vi "State_Machine.vi"(8 "error in (no error)":errorcluster caption="entrée d'erreur (pas d'erreur)", 11 "Get_Voltage en entrée":refnum<class "P2056_ExitTestBench.lvclass">) -> (0 "error out":errorcluster caption="sortie d'erreur", 2 "Json_String":string, 3 "Get_Voltage en sortie":refnum<class "P2056_ExitTestBench.lvclass">)   [LabVIEW 2020, in "Library Test.lvlib" / "P2056_ExitTestBench.lvclass"]
uses:
  P2056_ExitTestBench.lvclass
  C:/Users/ngarcin/OneDrive - Altyor/Standard TB/Class/Test/P2056_Send_Command_UART/P2056_Send_Command_UART.lvclass
  C:/Users/ngarcin/OneDrive - Altyor/Standard TB/Class/Test/Test (Default)/Test (Default).lvclass
  Instrument/Instrument (Default)/Class Instrument (Default).lvclass
  P2056_ExitTestBench.lvclass/P2056_ExitTestBench.ctl
  P2056_Send_Command_UART/P2056_Send_Command_UART.lvclass
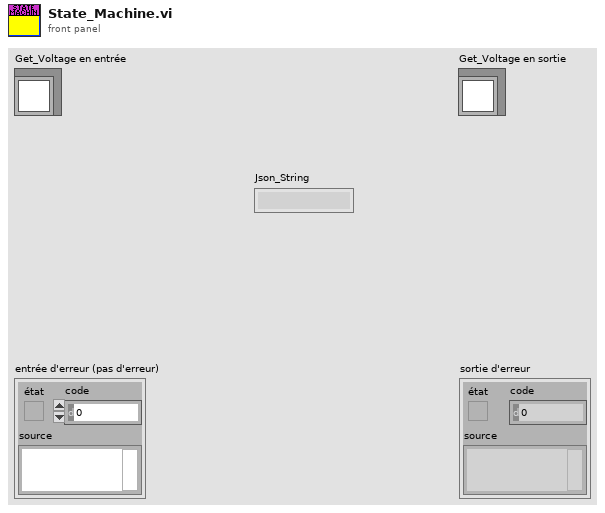
[diagram p1: front panel]
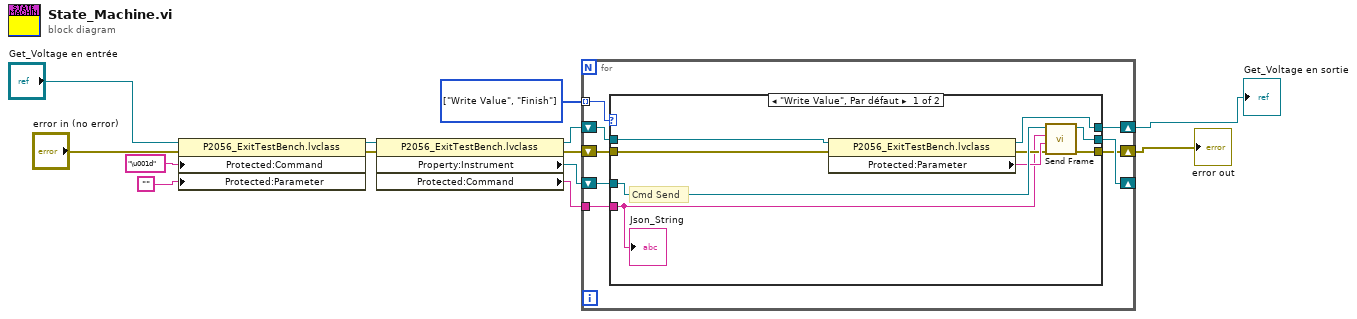
[diagram p0: block diagram]
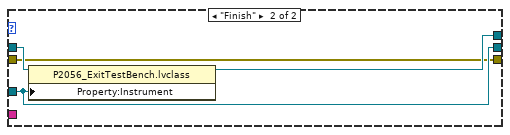
[diagram p2: hidden frame]
diagram:
  w9 = enum16{"Init", "Write Value", "Finish"}[] [enum."Write Value", enum."Finish"] items=["Init", "Write Value", "Finish"]
  n1 = property class="P2056_ExitTestBench.lvclass"(reference="Get_Voltage en entrée", error in="error in (no error)", "Protected:Command"="\u001d" ("chaîne"), "Protected:Parameter"="") -> (reference out=w4:refnum<class "P2056_ExitTestBench.lvclass">, error out=w3:errorcluster)
  n2 = property class="P2056_ExitTestBench.lvclass"(reference=w4, error in=w3) -> (reference out=w7:refnum<class "P2056_ExitTestBench.lvclass">, error out=w6:errorcluster, "Property:Instrument"=w8:refnum<class "Class Instrument (Default).lvclass">, "Protected:Command"=w5:string)
  n3 = for {
    tunnel: w9 -> [w21] mode=indexing
    shift-right: [w19] -> _
    shift-left: w8 -> [w20]
    shift-right: [w17] -> w1
    shift-left: w7 -> [w18]
    shift-right: [w15] -> w2
    shift-left: w6 -> [w16]
    tunnel: w5 -> [w14]
    n4 = case shown="\"Write Value\", Par défaut" w21 {
      tunnel: w20 -> [w28 w32]
      tunnel: [w29 w32] -> w19
      tunnel: w18 -> [w27 w34]
      tunnel: [w26 w33] -> w17
      tunnel: w16 -> [w24 w31]
      tunnel: [w30 w31] -> w15
      tunnel: w14 -> [w22 _]
      frame "Write Value", Default {
        # "Cmd Send"
        n5 = property class="P2056_ExitTestBench.lvclass"(reference=w27, error in=w24) -> (reference out=w26:refnum<class "P2056_ExitTestBench.lvclass">, error out=w23:errorcluster, "Protected:Parameter"=w25:string)
        n6 = call "Send Frame.vi"("entrée d'erreur (pas d'erreur)"=w23, "Parameter"=w25, "Cmd"=w22, "Class Instrument (Default) en entrée"=w28) -> ("sortie d'erreur"=w30:errorcluster, "Class Instrument (Default) en sortie"=w29:refnum<class "Class Instrument (Default).lvclass">)  [unwired: 6 in]
        "Json_String" <- w22
      }
      frame "Finish" {
        n7 = property class="P2056_ExitTestBench.lvclass"(reference=w34, "Property:Instrument"=w32) -> (reference out=w33:refnum<class "P2056_ExitTestBench.lvclass">)  [unwired: 1 in, 1 out]
      }
    }
  }
  "error out" <- w2
  "Get_Voltage en sortie" <- w1
